vi "kalibrace.vi"() -> ()   [LabVIEW 2024]
uses:
  <vilib>/Analysis/6fits.llb/Curve Fitting Criteria.ctl
  <vilib>/Analysis/baseanly.llb/Mean (DBL).vi
  <instrlib>/EFmeter/Public/Data/Read (Single Point).vi
  <instrlib>/EFmeter/EFmeter.lvlib
  <vilib>/Analysis/NI_AALBase.lvlib
  <vilib>/Analysis/NI_AALPro.lvlib
panel:
  in  "VISA EFmeter":refnum<visa-resource-name>
  in  "file path (use dialog)":path
  out "Polynomial Coefficients":dbl[](array[numeric])
  in  "Prumerovani":bool
  in  "Vzorku na krokù":u16 max=100 step=1
  in  "Reálná hodnota vstupní veličiny":dbl
  in  "Combo Box":string(combo)="VOLT"
  in  "Ring":u16(ring)=1 items=["CH2"=2, "CH1"=1]
  out "XY Graph 2":cluster{"X":dbl[], "Y":dbl[]}[](graph)
  in  "Clear":bool
  in  "Uložit data":bool
  in  "vyh\nVyhodnotit":bool
  in  "Další":bool caption="OK Button"
  in  "Start":bool
  in  "stop":bool
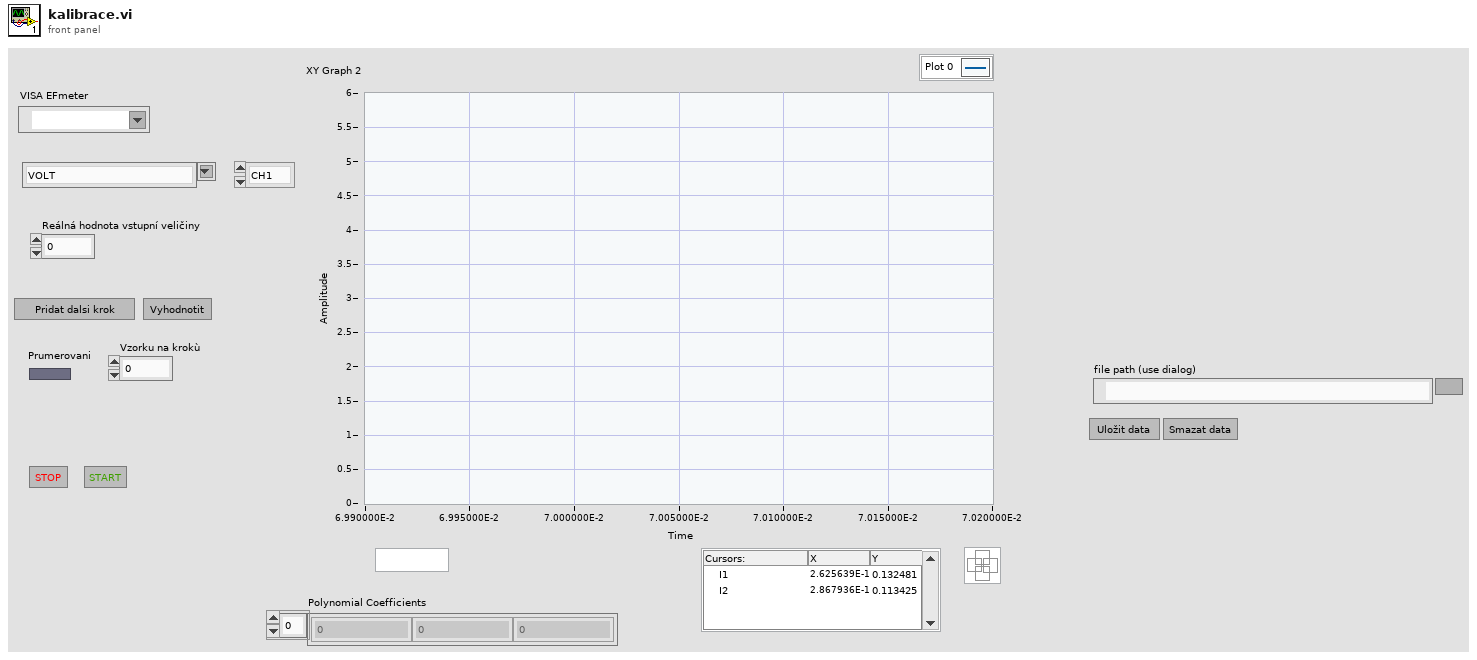
[diagram p1: front panel]
types:
  T1 = enum16{"init", "wait", "graph", "meas", "change_load", "init_measurment", "save", "clear"}
  T2 = enum16{"open", "replace", "create", "open or create", "replace or create", "replace or create with confirmation"}
  T3 = typedef "NI_AALPro.lvlib/Curve Fitting Criteria.ctl" = u16
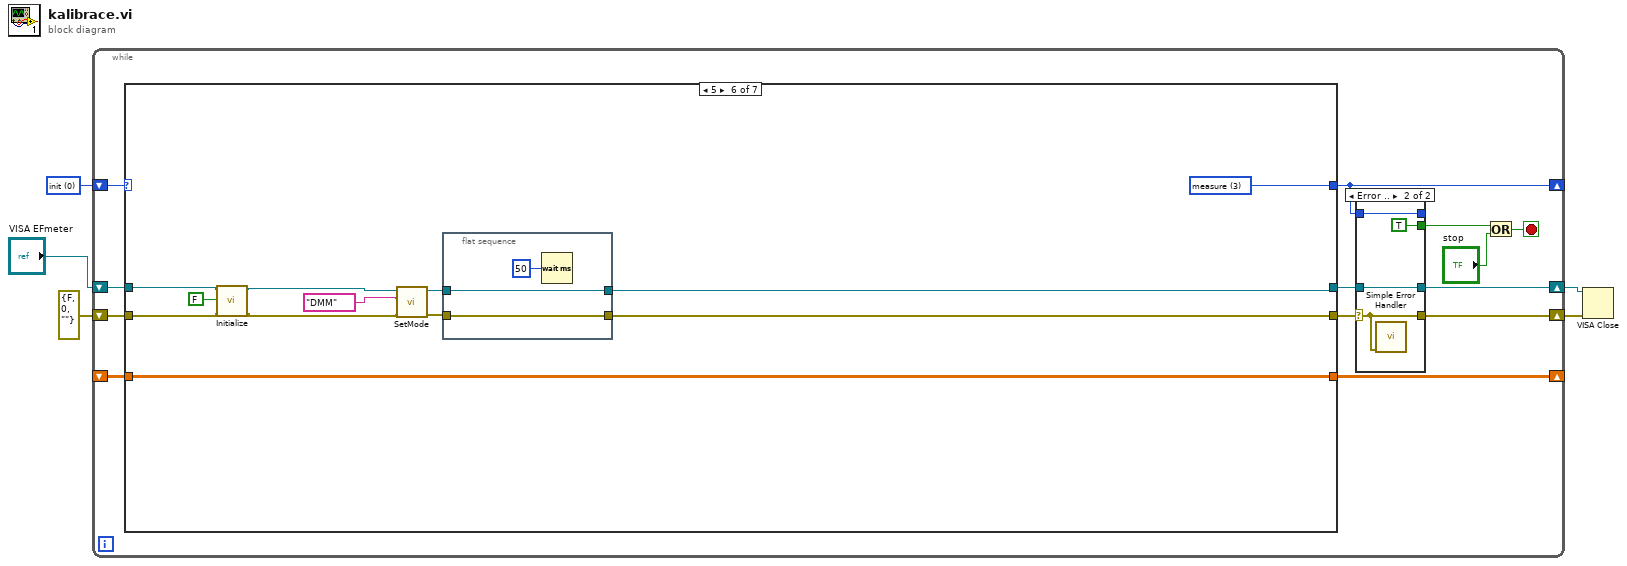
[diagram p0: block diagram]
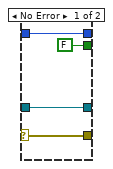
[diagram p2: hidden frame]
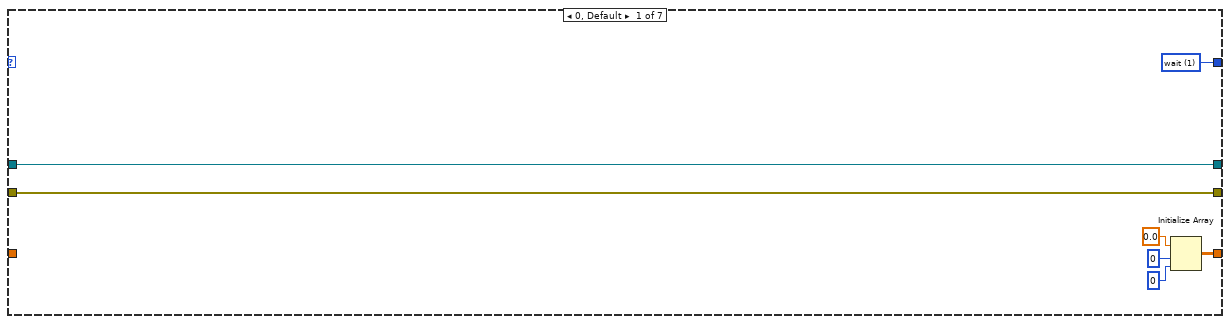
[diagram p3: hidden frame]
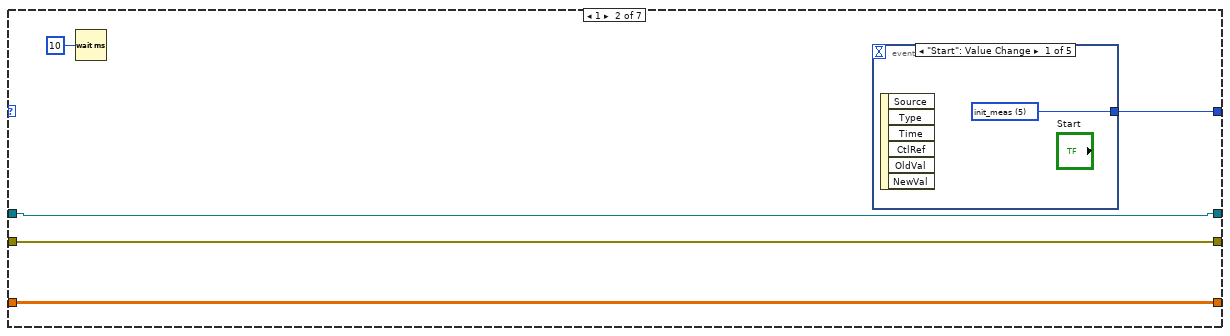
[diagram p4: hidden frame]
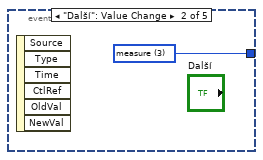
[diagram p5: hidden frame]
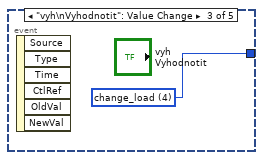
[diagram p6: hidden frame]
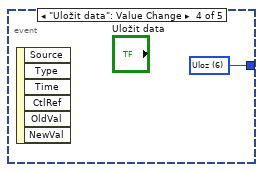
[diagram p7: hidden frame]
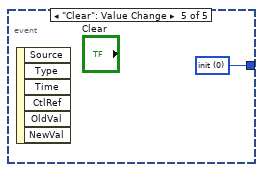
[diagram p8: hidden frame]
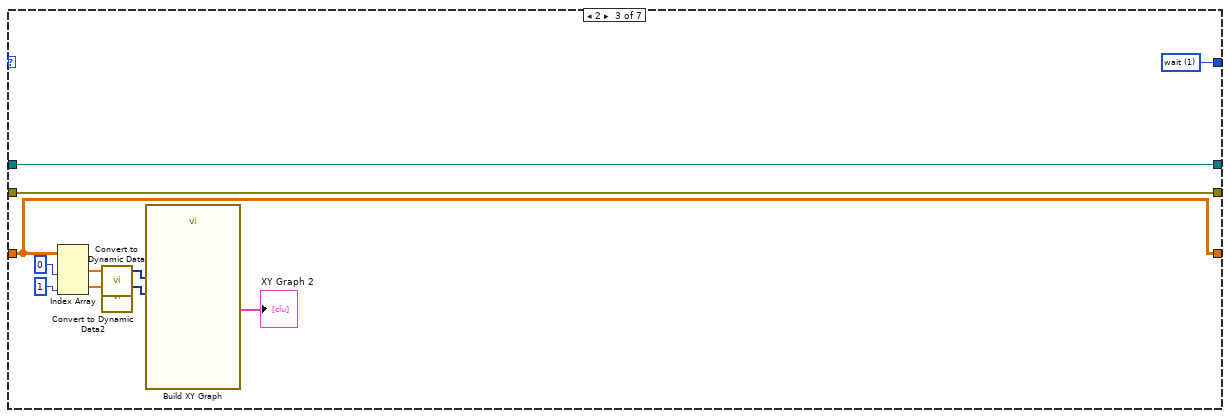
[diagram p9: hidden frame]
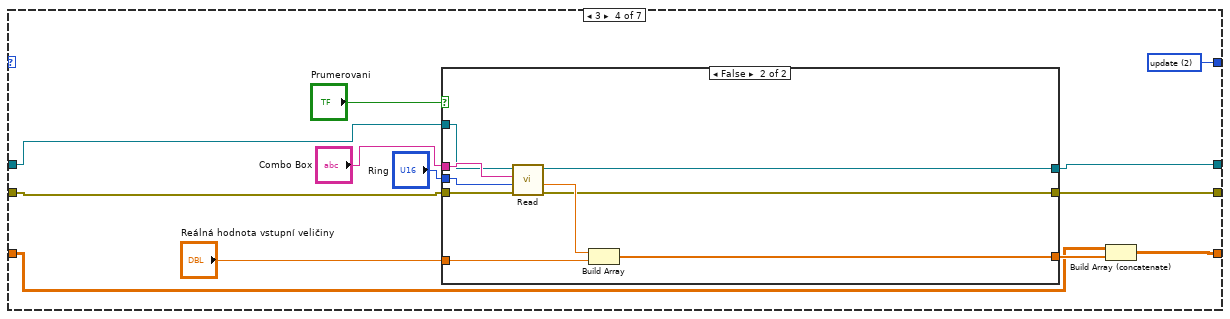
[diagram p10: hidden frame]
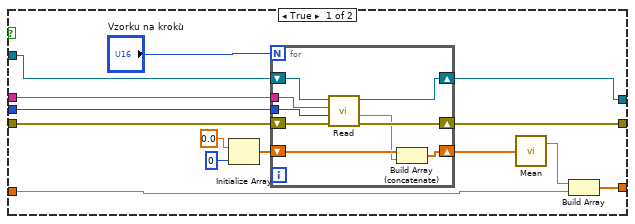
[diagram p11: hidden frame]
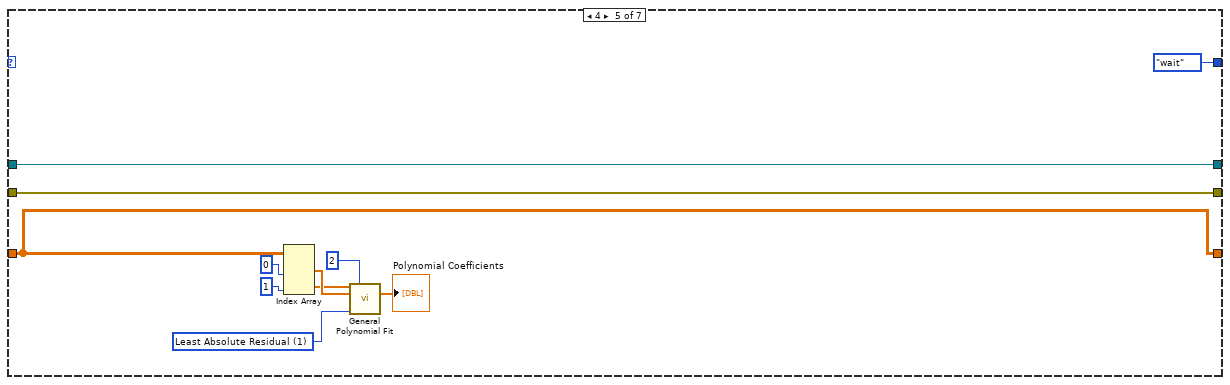
[diagram p12: hidden frame]
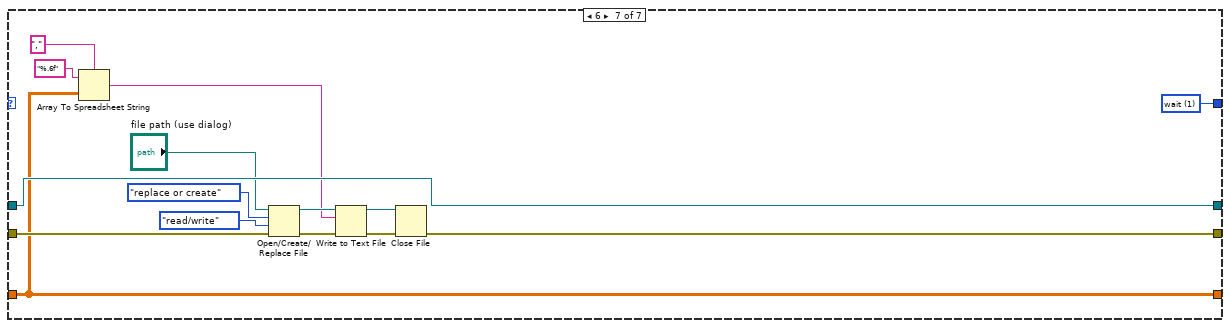
[diagram p13: hidden frame]
diagram:
  w5 = u16 0 items=["init", "wait", "update", "measure", "change_load", "init_meas", "Uloz", "clear"]
  n1 = while {
    shift-right: [w18] -> _
    shift-left: _ -> [w6]
    shift-right: [w14] -> _
    shift-left: w5 -> [w17]
    shift-right: [w11] -> w2
    shift-left: "VISA EFmeter" -> [w16]
    shift-right: [w10] -> w1
    shift-left: errorcluster {"status"=FALSE, "code"=0, "source"=""} ("error in (no error)") -> [w15]
    stop <- w8 stop-if-true
    n2 = case shown="5" w17 {
      tunnel: [w31 w34 w44 w66 w99 w118 w125] -> w18
      tunnel: [w30 w38 w45 w64 T1."wait" w121 w133] -> w14
      tunnel: [w27 w36 w46 w60 w107 w119 w129] -> w13
      tunnel: [w28 w37 w47 w61 w109 w120 w139] -> w12
      tunnel: w16 -> [w28 w37 w47 w63 w109 w116 w139]
      tunnel: w15 -> [w27 w36 w46 w62 w107 w115 w135]
      tunnel: w6 -> [_ w34 w44 w57 w99 w118 w125]
      frame 0, Default {
        w30 = u16 1 items=["init", "wait", "update", "measure"]
        n3 = Initialize Array(0.0 ("element"), 0 ("dimension size"), 0 ("dimension size")) -> (w31:dbl[][])
      }
      frame 1 {
        n4 = Wait (ms)(milliseconds to wait=u32 10) -> ()  [unwired: 1 out]
        n5 = event shown="[0] \"Start\": Value Change" {
          selector: _ -> [_ _ _ _ _]
          dyn-events: _ -> [_ _ _ _ _]
          timeout: _ -> [_ _ _ _ _]
          tunnel: [w39 w40 w41 w42 w43] -> w38
          event "Start": Value Change {
            w39 = u16 5 items=["init", "wait", "update", "measure", "change_load", "init_meas"]
            n6 = event-data() -> ()  [unwired: 1 in, 6 out]
          }
          event "Další": Value Change {
            w40 = u16 3 items=["init", "wait", "update", "measure", "change_load", "init_meas", "Uloz", "clear"]
            n7 = event-data() -> ()  [unwired: 1 in, 6 out]
          }
          event "vyh\nVyhodnotit": Value Change {
            w41 = u16 4 items=["init", "wait", "update", "measure", "change_load", "init_meas", "Uloz", "clear"]
            n8 = event-data() -> ()  [unwired: 1 in, 6 out]
          }
          event "Uložit data": Value Change {
            w42 = u16 6 items=["init", "wait", "update", "measure", "change_load", "init_meas", "Uloz"]
            n9 = event-data() -> ()  [unwired: 1 in, 6 out]
          }
          event "Clear": Value Change {
            w43 = u16 0 items=["init", "wait", "update", "measure", "change_load", "init_meas", "Uloz", "clear"]
            n10 = event-data() -> ()  [unwired: 1 in, 6 out]
          }
        }
      }
      frame 2 {
        w45 = u16 1 items=["init", "wait", "update", "measure"]
        n11 = Index Array(array=w44, index (col) #1=0 ("index (row)"), index (col) #2=1 ("index (row)")) -> (element #1=w54:dbl[], element #2=w51:dbl[])  [unwired: 2 in]
        n12 = call "Convert to Dynamic Data"("Array"=w54) -> ("Dynamic Data Type"=w53:dynamicdata)  [unwired: 3 in]
        n13 = call "Convert to Dynamic Data2"("Array"=w51) -> ("Dynamic Data Type"=w52:dynamicdata)  [unwired: 3 in]
        n14 = call "Build XY Graph"("Y Input"=w52, "X Input"=w53) -> ("XY Graph"=→"XY Graph 2":cluster{"X":dbl[], "Y":dbl[]}[])  [unwired: 8 in, 1 out]
      }
      frame 3 {
        w64 = u16 2 items=["init", "wait", "update", "measure"]
        n15 = case shown="False" "Prumerovani" {
          tunnel: [w73 w98] -> w65
          tunnel: w63 -> [w76 w93]
          tunnel: w62 -> [w75 w96]
          tunnel: [w72 w92] -> w61
          tunnel: [w71 w90] -> w60
          tunnel: "Reálná hodnota vstupní veličiny" -> [w69 w97]
          tunnel: "Combo Box" -> [w68 w94]
          tunnel: "Ring" -> [w67 w95]
          frame True {
            n16 = Initialize Array(0.0 ("element"), 0 ("dimension size")) -> (w77:dbl[])
            n17 = for {
              N: "Vzorku na krokù" -> [_]
              shift-right: [w81] -> w72
              shift-left: w76 -> [w84]
              shift-right: [w83] -> w71
              shift-left: w75 -> [w87]
              shift-right: [w88] -> w70
              shift-left: w77 -> [w89]
              tunnel: w68 -> [w86]
              tunnel: w67 -> [w85]
              n18 = call-poly <instrlib>:"Read.vi"("error in (no error)"=w87, "Ring"=w85, "Combo Box"=w86, "VISA resource name"=w84) -> ("error out"=w83:errorcluster, "Measurement"=w82:dbl, "VISA resource name out"=w81:refnum<visa-resource-name>)  [unwired: 5 in]
              n19 = Build Array (concatenate)(w89, w82) -> (w88:dbl[])
            }
            n20 = call-poly <vilib>:"Mean.vi"("X"=w70) -> ("mean"=w74:dbl)  [unwired: 1 out]
            n21 = Build Array(w74, w69) -> (w73:dbl[])
          }
          frame False {
            n22 = call-poly <instrlib>:"Read.vi"("error in (no error)"=w96, "Ring"=w95, "Combo Box"=w94, "VISA resource name"=w93) -> ("error out"=w90:errorcluster, "Measurement"=w91:dbl, "VISA resource name out"=w92:refnum<visa-resource-name>)  [unwired: 5 in]
            n23 = Build Array(w91, w97) -> (w98:dbl[])
          }
        }
        n24 = Build Array (concatenate)(w57, w65) -> (w66:dbl[][])
      }
      frame 4 {
        w100 = T3 1 items=["Least Square", "Least Absolute Residual", "Bisquare"] ("method")
        n25 = Index Array(array=w99, index (col) #1=0 ("disabled index (col)"), index (col) #2=1 ("disabled index (col)")) -> (element #1=w103:dbl[], element #2=w102:dbl[])  [unwired: 2 in]
        n26 = call <vilib>:"General Polynomial Fit.vi"("Y"=w102, "polynomial order"=2, "X"=w103, "method"=w100) -> ("Polynomial Coefficients"=→"Polynomial Coefficients":dbl[])  [unwired: 8 in, 3 out]
      }
      frame 5 {
        w121 = u16 3 items=["init", "wait", "update", "measure", "change_load", "init_meas"]
        n27 = call <instrlib>:"Initialize.vi"("error in (no error)"=w115, "ID Query (True)"=FALSE, "VISA resource name"=w116) -> ("error out"=w112:errorcluster, "VISA resource name out"=w110:refnum<visa-resource-name>)  [unwired: 7 in]
        n28 = call <instrlib>:"SetMode.vi"("error in (no error)"=w112, "Combo Box"="DMM", "VISA resource name"=w110) -> ("error out"=w113:errorcluster, "VISA resource name out"=w114:refnum<visa-resource-name>)  [unwired: 7 in]
        n29 = flat-sequence {
          tunnel: [w123] -> w120
          tunnel: w114 -> [w123]
          tunnel: w113 -> [w122]
          tunnel: [w122] -> w119
          frame #0 {
            n30 = Wait (ms)(milliseconds to wait=u32 50) -> ()  [unwired: 1 out]
          }
        }
      }
      frame 6 {
        w133 = u16 1 items=["init", "wait", "update", "measure", "change_load", "init_meas"]
        n31 = Array To Spreadsheet String(delimiter (Tab)=",", array=w125, 3:"%.6f" ("format string")) -> (spreadsheet string=w126:string)
        n32 = Open/Create/Replace File(file path (use dialog)="file path (use dialog)", error in=w135, operation (0:open)=T2."replace or create", access (0:read/write)=enum16{"read/write", "read-only", "write-only"}."read/write") -> (refnum out=w128:refnum<file>, error out=w131:errorcluster)  [unwired: 2 in, 1 out]
        n33 = Write to Text File(file (use dialog)=w128, text=w126, error in=w131) -> (refnum out=w127:refnum<file>, error out=w130:errorcluster)  [unwired: 1 in, 1 out]
        n34 = Close File(refnum=w127, error in=w130) -> (error out=w129:errorcluster)  [unwired: 1 out]
      }
    }
    n35 = case shown="Error .." w13 {
      selector: w13 -> [w20 w23]
      tunnel: w14 -> [w22 w25]
      tunnel: [w22 w25] -> _
      tunnel: w12 -> [w21 w26]
      tunnel: [w21 w26] -> w11
      tunnel: [w20 w23] -> w10
      tunnel: [FALSE TRUE] -> w7
      frame No Error {
      }
      frame Error {
        n36 = call <vilib>:"Simple Error Handler.vi"("error in (no error)"=w23) -> ()  [unwired: 4 in, 5 out]
      }
    }
    n37 = Or(x=w7, y="stop") -> (x .or. y?=w8:bool)
  }
  n38 = VISA Close(VISA resource name=w2, error in (no error)=w1) -> ()  [unwired: 1 out]
